vi "Simulator_0720.vi"() -> ()   [LabVIEW 2017]
doc: "This example demonstrates how to continuously acquire buffered voltage measurements using a DAQmx device.\n\nFor instructions on how to connect your signals to the DAQ device, refer to your device documentation."
uses:
  <vilib>/Utility/error.llb/DialogType.ctl
  <vilib>/DAQmx/read.llb/DAQmx Read (Analog 1D Wfm NChan NSamp).vi
  <vilib>/DAQmx/configure/task.llb/DAQmx Configure Logging (TDMS).vi
  <vilib>/express/express shared/transition.llb/Dynamic To Waveform Array.vi
  <vilib>/express/express arith-compare/Formula/Block/exnFormulaBlock how many pts in the wave.vi
  <vilib>/express/express shared/ex_Modify Signal Name.vi
  <vilib>/express/express shared/transition.llb/Waveform Array To Dynamic.vi
  <vilib>/measure/maspectr.llb/FFT Power Spectrum and PSD for N Chan.vi
  <vilib>/DAQmx/miscellaneous.llb/DAQmx Fill In Error Info.vi
  <vilib>/express/express arith-compare/Formula/XNode/ExpressFormulaBlockNode.xnode
  <vilib>/measure/NI_MAPro.lvlib
  SetupDAQ.vi
panel:
  out "2.5HZ-Step":dynamicdata(graph)
  in  "동작 라벨":T1(radio)
  in  "Sensor C Channel 2":tag="Dev2/ai0"
  in  "Sensor D Channel 2":tag="Dev2/ai1"
  in  "Terminal config 2":i32(ring)=10083 items=["default"=-1, "RSE"=10083, "NRSE"=10078, "Differential"=10106, "Pseudodifferential"=12529]
  out "55-65(A)":dynamicdata(graph)
  out "10-20(A)":dynamicdata(graph)
  out "Original Signal":waveform(dbl)[](graph)
  out "A,B Filtering Signal":dynamicdata(graph)
  out "Sensor A Raw 5":dynamicdata(graph)
  in  "number of averages":u32=1
  out "Power Spectrum / PSD":cluster{"f0":dbl, "df":dbl, "magnitude":dbl[]}[](graph)
  out "detected amplitudes 2":dbl(graph)=1.1331379876254155
  out "detected frequencies 2":dbl(graph)
  out "detected frequencies":dbl[](array[numeric])=[60.0, 60.0]
  out "detected amplitudes":dbl[](array[numeric])=[1.1331379876254155, 0.40633237156802526]
  out "Raw Signal 2":waveform(dbl)[](graph)
  out "Raw Signal":waveform(dbl)[](graph)
  in  "TDMS File Path":path
  in  "Logging Mode":i32(ring)=10231 items=["Off"=10231, "Log and Read"=15842]
  in  "Sensor B Channel":tag="Dev2/ai1"
  in  "Sensor A Channel":tag="Dev2/ai0"
  in  "Terminal config":i32(ring)=10083 items=["default"=-1, "RSE"=10083, "NRSE"=10078, "Differential"=10106, "Pseudodifferential"=12529]
  in  "rate":dbl=5000.0
  out "FFT Power Spectrum":cluster{"f0":dbl, "df":dbl, "magnitude":dbl[]}[](graph)
  in  "Stop":bool
  in  "Number of Samples":i32=100
  # "Channel Settings"
  # "Logging Settings"
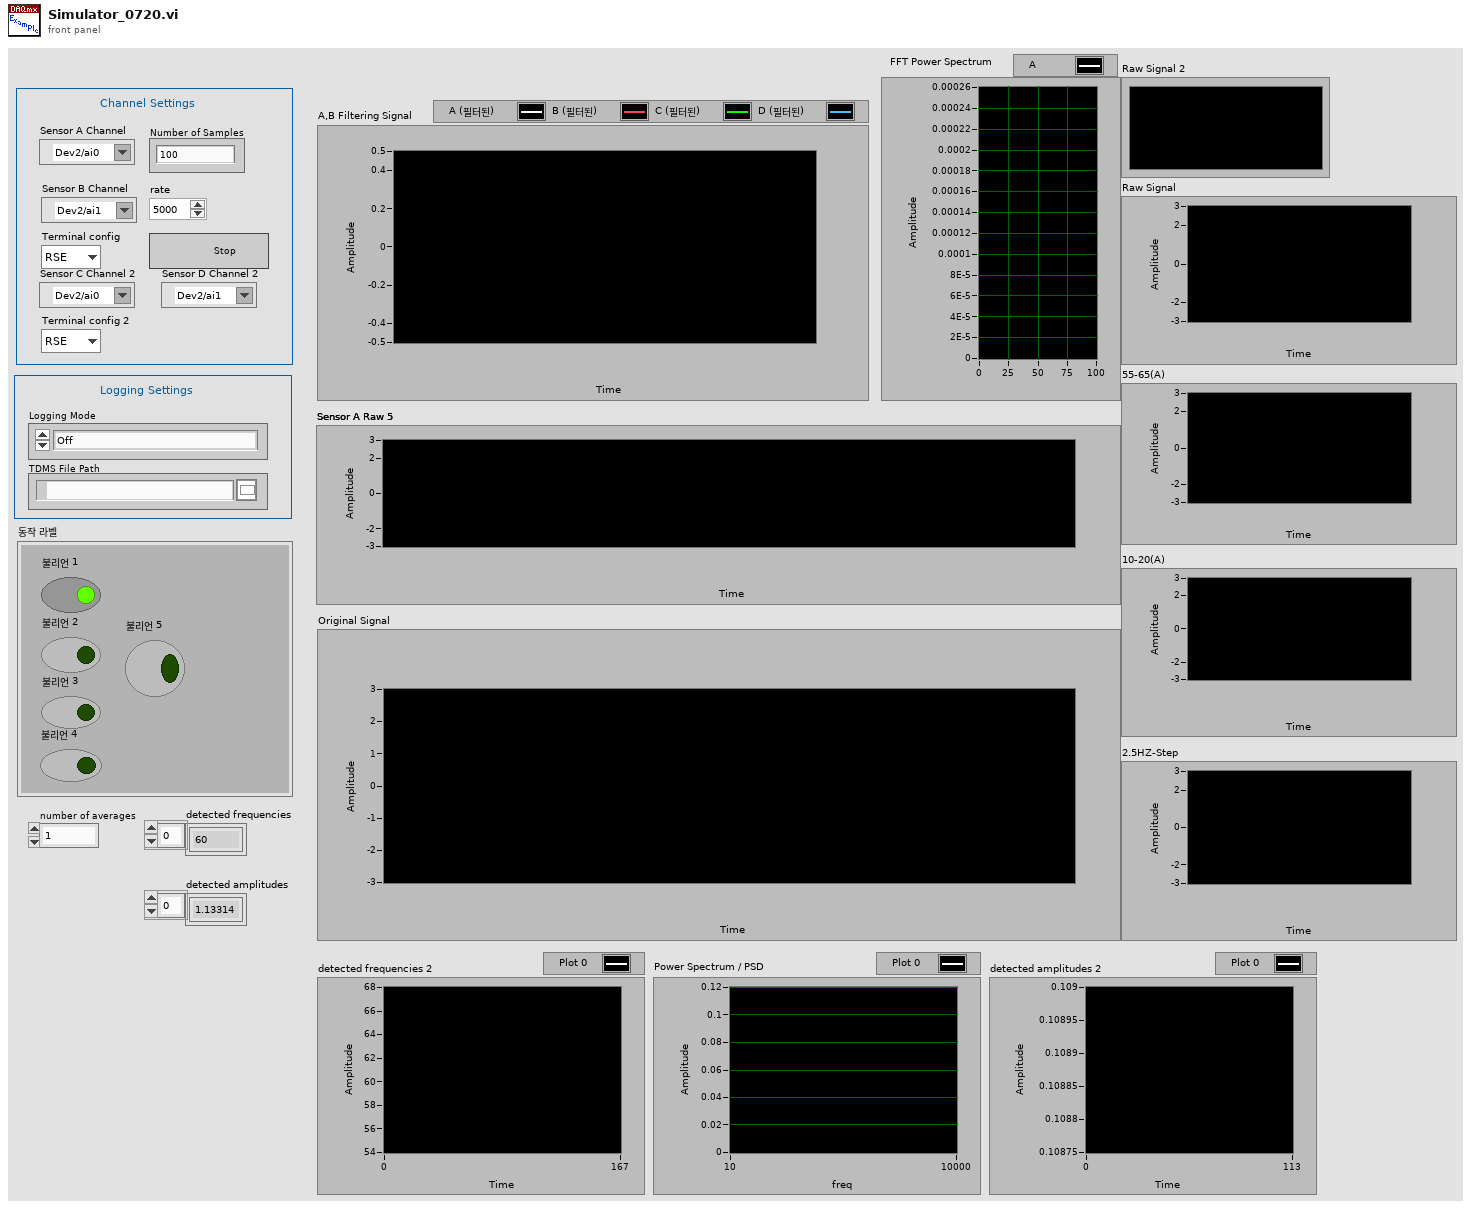
[diagram p1: front panel]
types:
  T1 = enum32{"불리언 1", "불리언 2", "불리언 3", "불리언 4", "불리언 5"}
  T2 = typedef "DialogType.ctl" = u16
  T3 = cluster{"averaging mode":enum16{"No averaging", "Vector averaging", "RMS averaging", "Peak hold"}, "weighting mode":enum16{"Linear", "Exponential"}, "number of averages":u32}
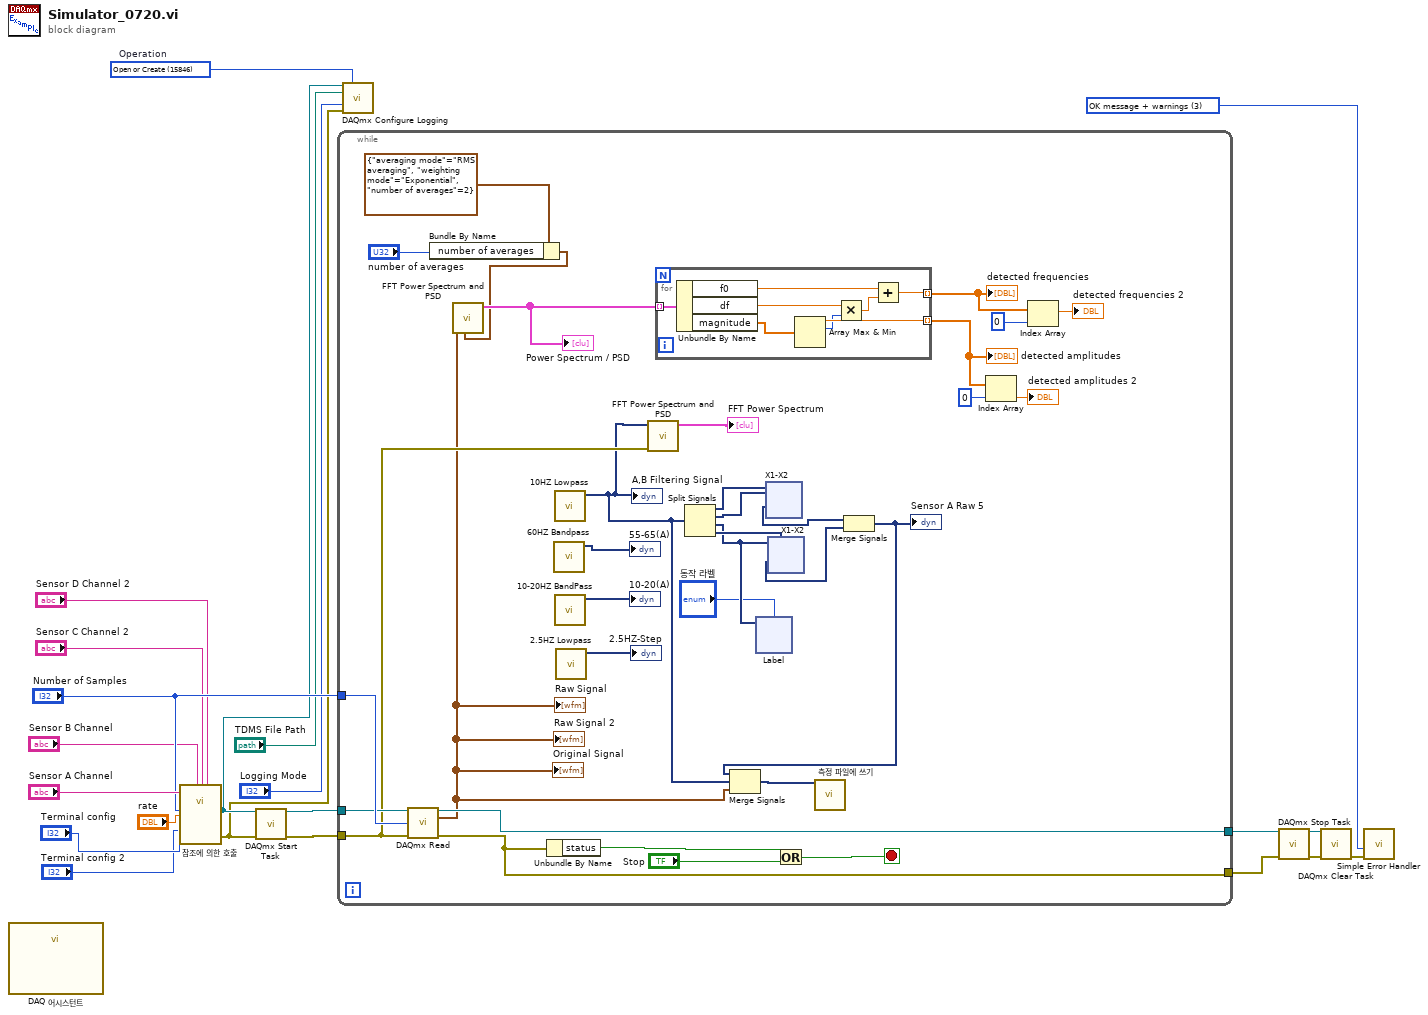
[diagram p0: block diagram]
diagram:
  w10 = 15846 items=["Open"=10437, "Open or Create"=15846, "Create or Replace"=15847, "Create"=15848]  # Operation
  w14 = T2 3 items=["no dialog", "OK message", "continue or stop message", "OK message + warnings", "continue/stop + warnings"] ("type of dialog (OK msg:1)")
  n1 = call "DAQ 어시스턴트"() -> ()  [unwired: 12 in]
  n2 = call-by-ref "참조에 의한 호출"("number of samples"="Number of Samples", "rate"="rate", "input terminal configuration"="Terminal config", "input terminal configuration 2"="Terminal config 2", "physical channel"="Sensor A Channel", "physical channel 2"="Sensor B Channel", "physical channel 3"="Sensor C Channel 2", "physical channel 4"="Sensor D Channel 2") -> ("task out"=w7:refnum<k21>, "error out"=w6:errorcluster)  [unwired: 12 in, 2 out]
  n3 = call <vilib>:"DAQmx Start Task.vi"("task/channels in"=w7, "error in"=w6) -> ("task out"=w21:refnum<k21>, "error out"=w20:errorcluster)  [unwired: 12 in]
  n4 = while "While 루프" {
    tunnel: w21 -> [w49]
    tunnel: w20 -> [w48]
    tunnel: [w54] -> w18
    tunnel: [w52] -> w17
    tunnel: "Number of Samples" -> [w50]
    stop <- w51 stop-if-true
    n5 = call-poly <vilib>:"DAQmx Read.vi"("task/channels in"=w49, "number of samples per channel"=w50, "error in"=w48) -> ("task out"=w54:refnum<k21>, "data"=w26:waveform(dbl)[], "error out"=w52:errorcluster)  [unwired: 10 in]
    "Raw Signal" <- w26
    "Raw Signal 2" <- w26
    "Original Signal" <- w26
    n6 = Bundle By Name ("이름으로 묶기")(cluster=T3 {"averaging mode"=enum."RMS averaging", "weighting mode"=enum."Exponential", "number of averages"=2} ("averaging parameters"), "number of averages"="number of averages") -> (w22:T3)
    n7 = call-poly <vilib>:"FFT Power Spectrum and PSD.vi"("averaging parameters"=w22, "time signals"=w26) -> ("Power Spectrum / PSD"=w24:cluster{"f0":dbl, "df":dbl, "magnitude":dbl[]}[])  [unwired: 6 in, 3 out]
    "Power Spectrum / PSD" <- w24
    n8 = Unbundle By Name(w52) -> ("status"=w39:bool)
    n9 = call "60HZ Bandpass"() -> ("Filtered Signal"=→"55-65(A)":dynamicdata)  [unwired: 10 in, 1 out]
    n10 = call "10HZ Lowpass"() -> ("Filtered Signal"=w28:dynamicdata)  [unwired: 10 in, 1 out]
    "A,B Filtering Signal" <- w28
    n11 = call "10-20HZ BandPass"() -> ("Filtered Signal"=→"10-20(A)":dynamicdata)  [unwired: 10 in, 1 out]
    n12 = call "2.5HZ Lowpass"() -> ("Filtered Signal"=→"2.5HZ-Step":dynamicdata)  [unwired: 10 in, 1 out]
    n13 = call-poly <vilib>:"FFT Power Spectrum and PSD.vi"("error in (no error)"=w48, "time signals"=w28) -> ("Power Spectrum / PSD"=→"FFT Power Spectrum":cluster{"f0":dbl, "df":dbl, "magnitude":dbl[]}[])  [unwired: 6 in, 3 out]
    n14 = for {
      tunnel: w24 -> [w337] mode=indexing
      tunnel: [w340] -> w45 mode=indexing
      tunnel: [w338] -> w42 mode=indexing
      n15 = Unbundle By Name(w337) -> ("f0"=w333:dbl, "df"=w339:dbl, "magnitude"=w336:dbl[])
      n16 = Array Max & Min(array=w336) -> (max value=w340:dbl, max index (indices)=w335:i32)  [unwired: 2 out]
      n17 = Multiply(x=w339, y=w335) -> (x*y=w334:dbl)
      n18 = Add(x=w333, y=w334) -> (x+y=w338:dbl)
    }
    "detected amplitudes" <- w45
    "detected frequencies" <- w42
    n19 = Split Signals(w28) -> (w35:dynamicdata, w34:dynamicdata, w30:dynamicdata, w33:dynamicdata)  [unwired: 4 in]
    n20 = xnode "Label"("X1"=w30, "X2"="동작 라벨") -> ()  [unwired: 1 in, 2 out]
    n21 = xnode "X1-X2"("X1"=w35, "X2"=w34) -> ("결과"=w32:dynamicdata)  [unwired: 1 in, 1 out]
    n22 = xnode "X1-X2"("X1"=w30, "X2"=w33) -> ("결과"=w31:dynamicdata)  [unwired: 1 in, 1 out]
    n23 = Or(x=w39, y="Stop") -> (x .or. y?=w51:bool)
    n24 = Merge Signals(w32, w31) -> (w27:dynamicdata)
    "Sensor A Raw 5" <- w27
    n25 = Merge Signals(w27, w28, w26) -> (w25:dynamicdata)
    n26 = call "측정 파일에 쓰기"("Signals"=w25) -> ()  [unwired: 16 in, 3 out]
    n27 = Index Array(array=w45, index=0) -> (element=→"detected amplitudes 2":dbl)
    n28 = Index Array(array=w42, index=0) -> (element=→"detected frequencies 2":dbl)
  }
  n29 = call-poly <vilib>:"DAQmx Configure Logging.vi"("task/channels in"=w7, "operation"=w10, "file path"="TDMS File Path", "logging mode"="Logging Mode", "error in"=w6) -> ()  [unwired: 9 in, 2 out]
  n30 = call <vilib>:"DAQmx Stop Task.vi"("task/channels in"=w18, "error in"=w17) -> ("task out"=w15:refnum<k21>, "error out"=w16:errorcluster)  [unwired: 12 in]
  n31 = call <vilib>:"DAQmx Clear Task.vi"("task in"=w15, "error in"=w16) -> ("error out"=w19:errorcluster)  [unwired: 13 in]
  n32 = call <vilib>:"Simple Error Handler.vi"("type of dialog (OK msg:1)"=w14, "error in (no error)"=w19) -> ()  [unwired: 3 in, 5 out]
